vi "Query Int.vi"(8 "error in (no error)":errorcluster, 10 "write buffer":string, 11 "VISA resource name In":refnum<visa-resource-name>) -> (0 "error out":errorcluster, 2 "int":u32, 3 "VISA resource name out":refnum<visa-resource-name>)   [LabVIEW 2013, in "Newport 1830-C.lvlib"]
doc: "Reads the and unsigned 32-bit integer from the output buffer of the instrument."
uses:
  Newport 1830-C.lvlib
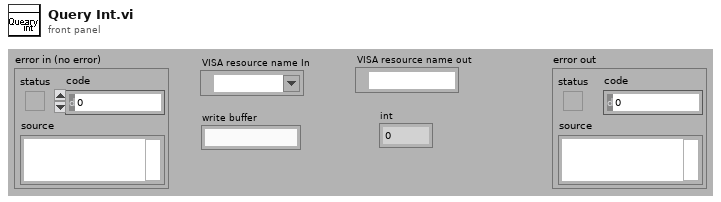
[diagram p1: front panel]
types:
  T1 = typedef "Semaphore RefNum" = refnum<k1>
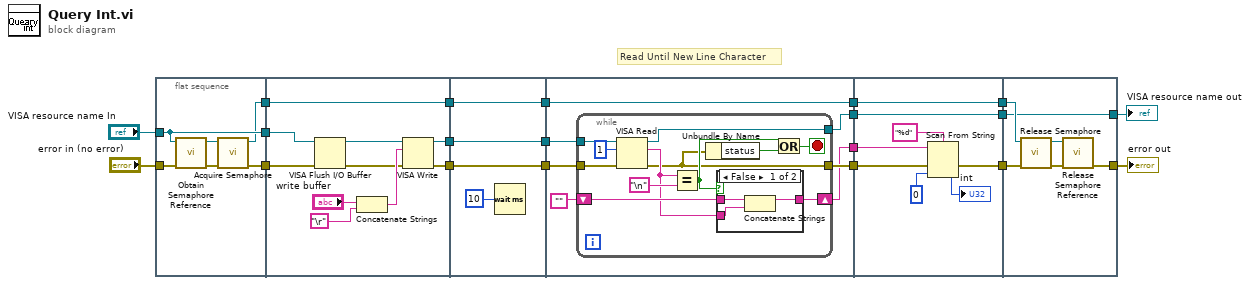
[diagram p0: block diagram]
diagram:
  # "Read Until New Line Character"
  n1 = flat-sequence {
    tunnel: "error in (no error)" -> [w26]
    tunnel: "VISA resource name In" -> [w22]
    tunnel: [w23] -> w18
    tunnel: [w22] -> w17
    tunnel: [w21] -> w9
    tunnel: w18 -> [w27]
    tunnel: w17 -> [w28]
    tunnel: [w36] -> w15
    tunnel: [w35] -> w13
    tunnel: [w34] -> w10
    tunnel: w9 -> [w34]
    tunnel: [w39] -> w16
    tunnel: w15 -> [w39]
    tunnel: [w38] -> w14
    tunnel: w13 -> [w38]
    tunnel: [w37] -> w11
    tunnel: w10 -> [w37]
    tunnel: w16 -> [w45]
    tunnel: w14 -> [w46]
    tunnel: [w47] -> w8
    tunnel: w11 -> [w47]
    tunnel: [w41] -> w6
    tunnel: [w44] -> w5
    tunnel: [w43] -> w1
    tunnel: w8 -> [w71]
    tunnel: [w71] -> w7
    tunnel: w6 -> [w68]
    tunnel: w5 -> [w67]
    tunnel: [w66] -> w4
    tunnel: [w65] -> w2
    tunnel: w1 -> [w65]
    tunnel: [w76] -> w12
    tunnel: w7 -> [w75]
    tunnel: w4 -> [w73]
    tunnel: [w72] -> w3
    tunnel: w2 -> [w72]
    frame #0 {
      n2 = call <vilib>:"Obtain Semaphore Reference.vi"("error in (no error)"=w26, "name (unnamed)"=w22) -> ("error out"=w24:errorcluster, "semaphore"=w25:T1)  [unwired: 3 in, 1 out]
      n3 = call <vilib>:"Acquire Semaphore.vi"("error in (no error)"=w24, "semaphore"=w25) -> ("error out"=w23:errorcluster, "semaphore out"=w21:T1)  [unwired: 3 in, 1 out]
    }
    frame #1 {
      n4 = VISA Flush I/O Buffer(VISA resource name=w28, error in (no error)=w27) -> (VISA resource name out=w29:refnum<visa-resource-name>, error out=w30:errorcluster)  [unwired: 1 in]
      n5 = Concatenate Strings("write buffer", "\r") -> (w31:string)
      n6 = VISA Write(VISA resource name=w29, write buffer=w31, error in (no error)=w30) -> (VISA resource name out=w35:refnum<visa-resource-name>, error out=w36:errorcluster)  [unwired: 1 out]
    }
    frame #2 {
      n7 = Wait (ms)(milliseconds to wait=u32 10) -> ()  [unwired: 1 out]
    }
    frame #3 {
      n8 = while {
        tunnel: w46 -> [w59]
        tunnel: w45 -> [w58]
        tunnel: [w49] -> w44
        tunnel: [w56] -> w43
        shift-right: [w54] -> w41
        shift-left: "" -> [w53]
        stop <- w51 stop-if-true
        n9 = VISA Read(VISA resource name=w59, byte count=u32 1, error in (no error)=w58) -> (VISA resource name out=w56:refnum<visa-resource-name>, read buffer=w52:string, error out=w49:errorcluster)  [unwired: 1 out]
        n10 = Equal?(x=w52, y="\n") -> (x = y?=w50:bool)
        n11 = Unbundle By Name(w49) -> ("status"=w48:bool)
        n12 = case shown="False" w50 {
          tunnel: [w62 w63] -> w54
          tunnel: w53 -> [w61 w63]
          tunnel: w52 -> [w60 _]
          frame False {
            n13 = Concatenate Strings(w61, w60) -> (w62:string)
          }
          frame True {
          }
        }
        n14 = Or(x=w50, y=w48) -> (x .or. y?=w51:bool)
      }
    }
    frame #4 {
      n15 = Scan From String(format string="%d", input string=w68, error in=w67, default 1=u32 0) -> (error out=w66:errorcluster, output 1=→"int":u32)  [unwired: 1 in, 2 out]
    }
    frame #5 {
      n16 = call <vilib>:"Release Semaphore.vi"("error in (no error)"=w73, "semaphore"=w75) -> ("error out"=w77:errorcluster, "semaphore out"=w74:T1)  [unwired: 4 in]
      n17 = call <vilib>:"Release Semaphore Reference.vi"("error in (no error)"=w77, "semaphore"=w74) -> ("error out"=w76:errorcluster)  [unwired: 8 in, 1 out]
    }
  }
  "error out" <- w12
  "VISA resource name out" <- w3
